vi "getDtFromXml.vi"(8 "error in (no error)":errorcluster, 10 "Xml":refnum<class "xmlNode.lvclass">, 11 "ScriptEvent in":refnum<class "ScriptEvent.lvclass">) -> (0 "error out":errorcluster, 2 "Xml out":refnum<class "xmlNode.lvclass">, 3 "ScriptEvent out":refnum<class "ScriptEvent.lvclass">)   [LabVIEW 2011, in "Tools.lvlib" / "Scripting.lvlib" / "ScriptEvent.lvclass"]
uses:
  ScriptEvent.lvclass
  xmlNode/xmlNode.lvclass
  ScriptEvent.lvclass/ScriptEvent.ctl
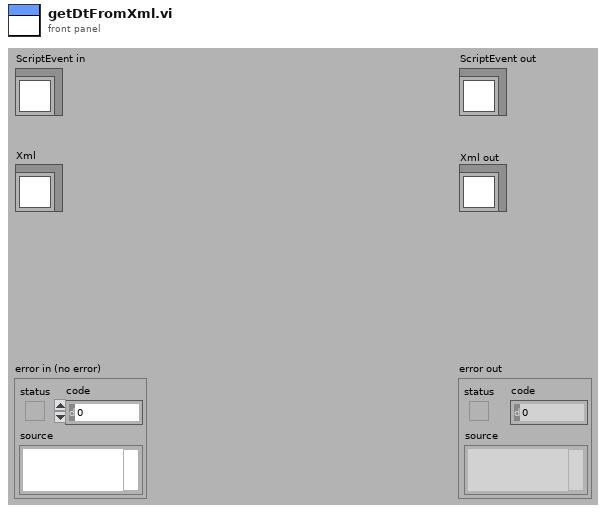
[diagram p1: front panel]
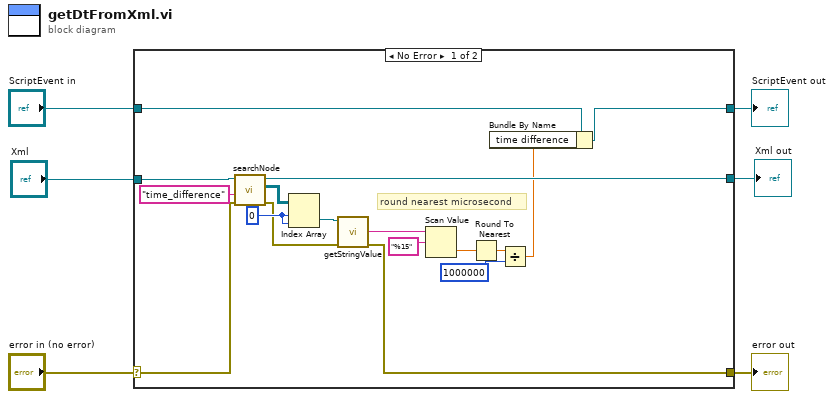
[diagram p0: block diagram]
diagram:
  n1 = case shown="No Error" "error in (no error)" {
    selector: "error in (no error)" -> [w12 w25]
    tunnel: [w13 w25] -> w5
    tunnel: [w15 w24] -> w3
    tunnel: "ScriptEvent in" -> [w16 w24]
    tunnel: "Xml" -> [w23 _]
    tunnel: [w14 _] -> w1
    frame No Error {
      w20 = 0
      # "round nearest microsecond"
      n2 = call-dynamic "searchNode.vi"("error in (no error)"=w12, "searchElementName"="time_difference", "xmlNode in"=w23) -> ("error out"=w11:errorcluster, "arrayXmlNodes"=w21:refnum<class "xmlNode.lvclass">[][], "xmlNode out"=w14:refnum<class "xmlNode.lvclass">)  [unwired: 6 in]
      n3 = Index Array(array=w21, index (row)=w20, index (col)=w20) -> (element=w19:refnum<class "xmlNode.lvclass">)
      n4 = call-dynamic "getStringValue.vi"("error in (no error)"=w11, "xmlNode.lvclass in"=w19) -> ("error out"=w13:errorcluster, "stringValue"=w18:string)  [unwired: 7 in, 1 out]
      n5 = Scan Value(string=w18, format string="%15") -> (value=w9:dbl)  [unwired: 1 in, 1 out]
      n6 = Round To Nearest(number=w9) -> (nearest integer value=w7:dbl)
      n7 = Divide(x=w7, y=1000000) -> (x/y=w8:dbl)
      n8 = Bundle By Name(cluster=w16, "time difference"=w8) -> (w15:refnum<class "ScriptEvent.lvclass">)
    }
    frame Error {
    }
  }
  "error out" <- w5
  "ScriptEvent out" <- w3
  "Xml out" <- w1
